vi "Find Matching Actual Value Channel.vi"(8 "error in (no error)":errorcluster, 11 "Desired item ref in":T1 format="%.0x") -> (0 "error out":errorcluster, 1 "Refs (desired first)":T1[](array[typedef]) format="%.0x", 2 "Actual item ref":T1 format="%.0x", 3 "Desired item ref out":T1 format="%.0x", 5 "found":bool, 7 "CH#":string)   [LabVIEW 2011, in "NI 272x Resistive Simulation Custom Device Configuration.lvlib"]
uses:
  NI 272x Resistive Simulation Custom Device Configuration.lvlib
  <vilib>/NI Veristand/Custom Device API/Custom Device Item Ref.ctl
  Globals/Names.vi
  <vilib>/NI Veristand/Custom Device API/Get Item Property (I32).vi
  <vilib>/NI Veristand/Custom Device API/Custom Device API.lvlib
  NI 272x Resistive Simulation Custom Device Shared.lvlib
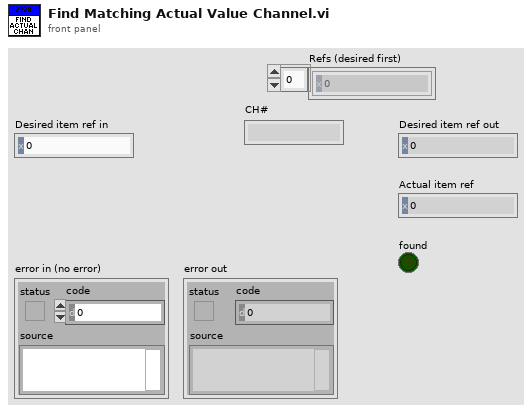
[diagram p1: front panel]
types:
  T1 = typedef "Custom Device API.lvlib/Custom Device Item Ref.ctl" = u64
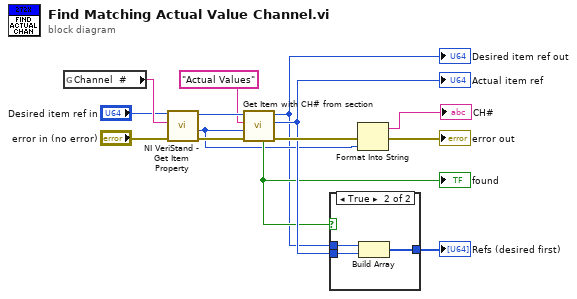
[diagram p0: block diagram]
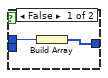
[diagram p2: hidden frame]
diagram:
  n1 = global read "Names.vi" "Channel  #"() -> (w11:string)
  n2 = call-poly <vilib>:"NI VeriStand - Get Item Property.vi"("error in (no error)"="error in (no error)", "Property Name"=w11, "Item Ref in"="Desired item ref in") -> ("error out"=w13:errorcluster, "Value"=w3:i32, "Item Ref out"=w12:T1)  [unwired: 5 in, 1 out]
  n3 = call "Get Item with CH# from section.vi"("error in (no error)"=w13, "CH#"=w3, "Section containing ch#"="Actual Values" ("Item Name"), "Item Ref in"=w12) -> ("error out"=w9:errorcluster, "Matching CH# item in Specified Section"=w5:T1, "Item Ref out"=w1:T1, "Found"=w4:bool)  [unwired: 4 in]
  "Desired item ref out" <- w1
  "found" <- w4
  "Actual item ref" <- w5
  n4 = case shown="True" w4 {
    tunnel: w1 -> [w16 w19]
    tunnel: w5 -> [_ w18]
    tunnel: [w15 w17] -> w10
    frame False {
      n5 = Build Array(w16) -> (w15:T1[])
    }
    frame True {
      n6 = Build Array(w19, w18) -> (w17:T1[])
    }
  }
  "Refs (desired first)" <- w10
  n7 = Format Into String(error in=w9, w3) -> (resulting string=→"CH#":string, error out=→"error out":errorcluster)  [unwired: 2 in]
